vi "导入参数设置3.0.vi"(0 "路径":path) -> (7 "输出":T1)   [LabVIEW 2016]
uses:
  <vilib>/Utility/config.llb/Read Key (String).vi
  <vilib>/Utility/config.llb/Read Key (Double).vi
  <vilib>/Utility/config.llb/NI_LVConfig.lvlib
panel:
  in  "ESC":bool
  in  "OK":bool
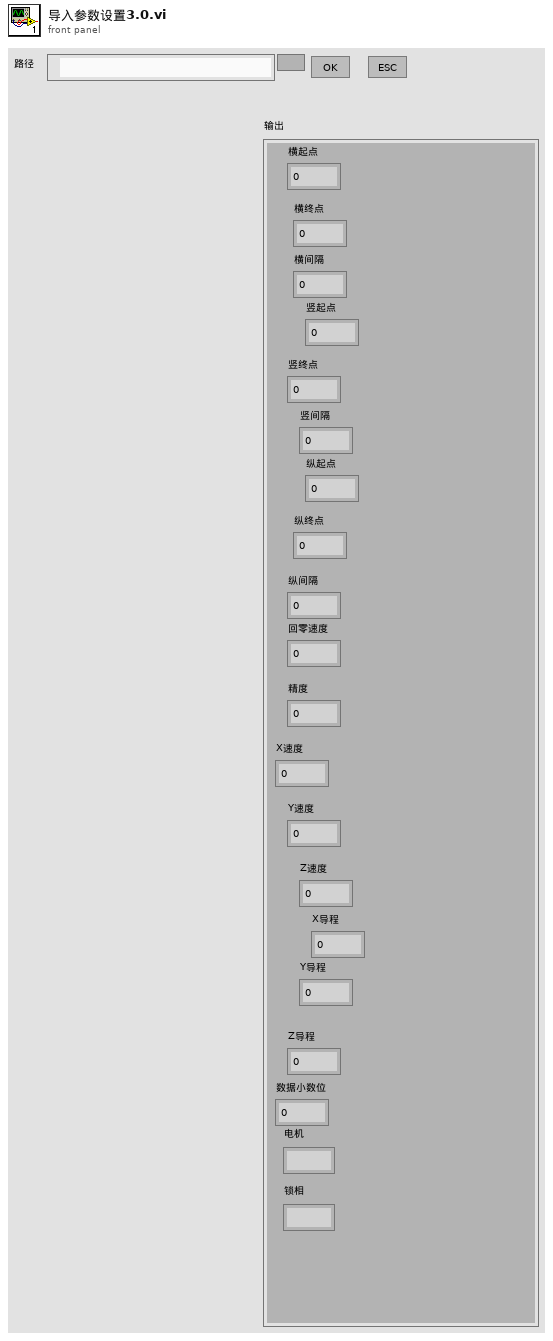
[diagram p1: front panel]
types:
  T1 = cluster{"横起点":dbl, "横终点":dbl, "横间隔":dbl, "竖起点":dbl, "竖终点":dbl, "竖间隔":dbl, "纵起点":dbl, "纵终点":dbl, "纵间隔":dbl, "回零速度":dbl, "精度":dbl, "X速度":dbl, "Y速度":dbl, "Z速度":dbl, "X导程":dbl, "Y导程":dbl, "Z导程":dbl, "数据小数位":dbl, "电机":string, "锁相":string}
  T2 = typedef "NI_LVConfig.lvlib/Config Data RefNum.ctl" = refnum<k1>
  T3 = cluster{"value":dbl, "value":dbl, "value":dbl, "value":dbl, "value":dbl, "value":dbl, "value":dbl, "value":dbl, "value":dbl, "value":dbl, "value":dbl, "value":dbl, "value":dbl, "value":dbl, "value":dbl, "value":dbl, "value":dbl, "value":dbl, "value":string, "value":string}
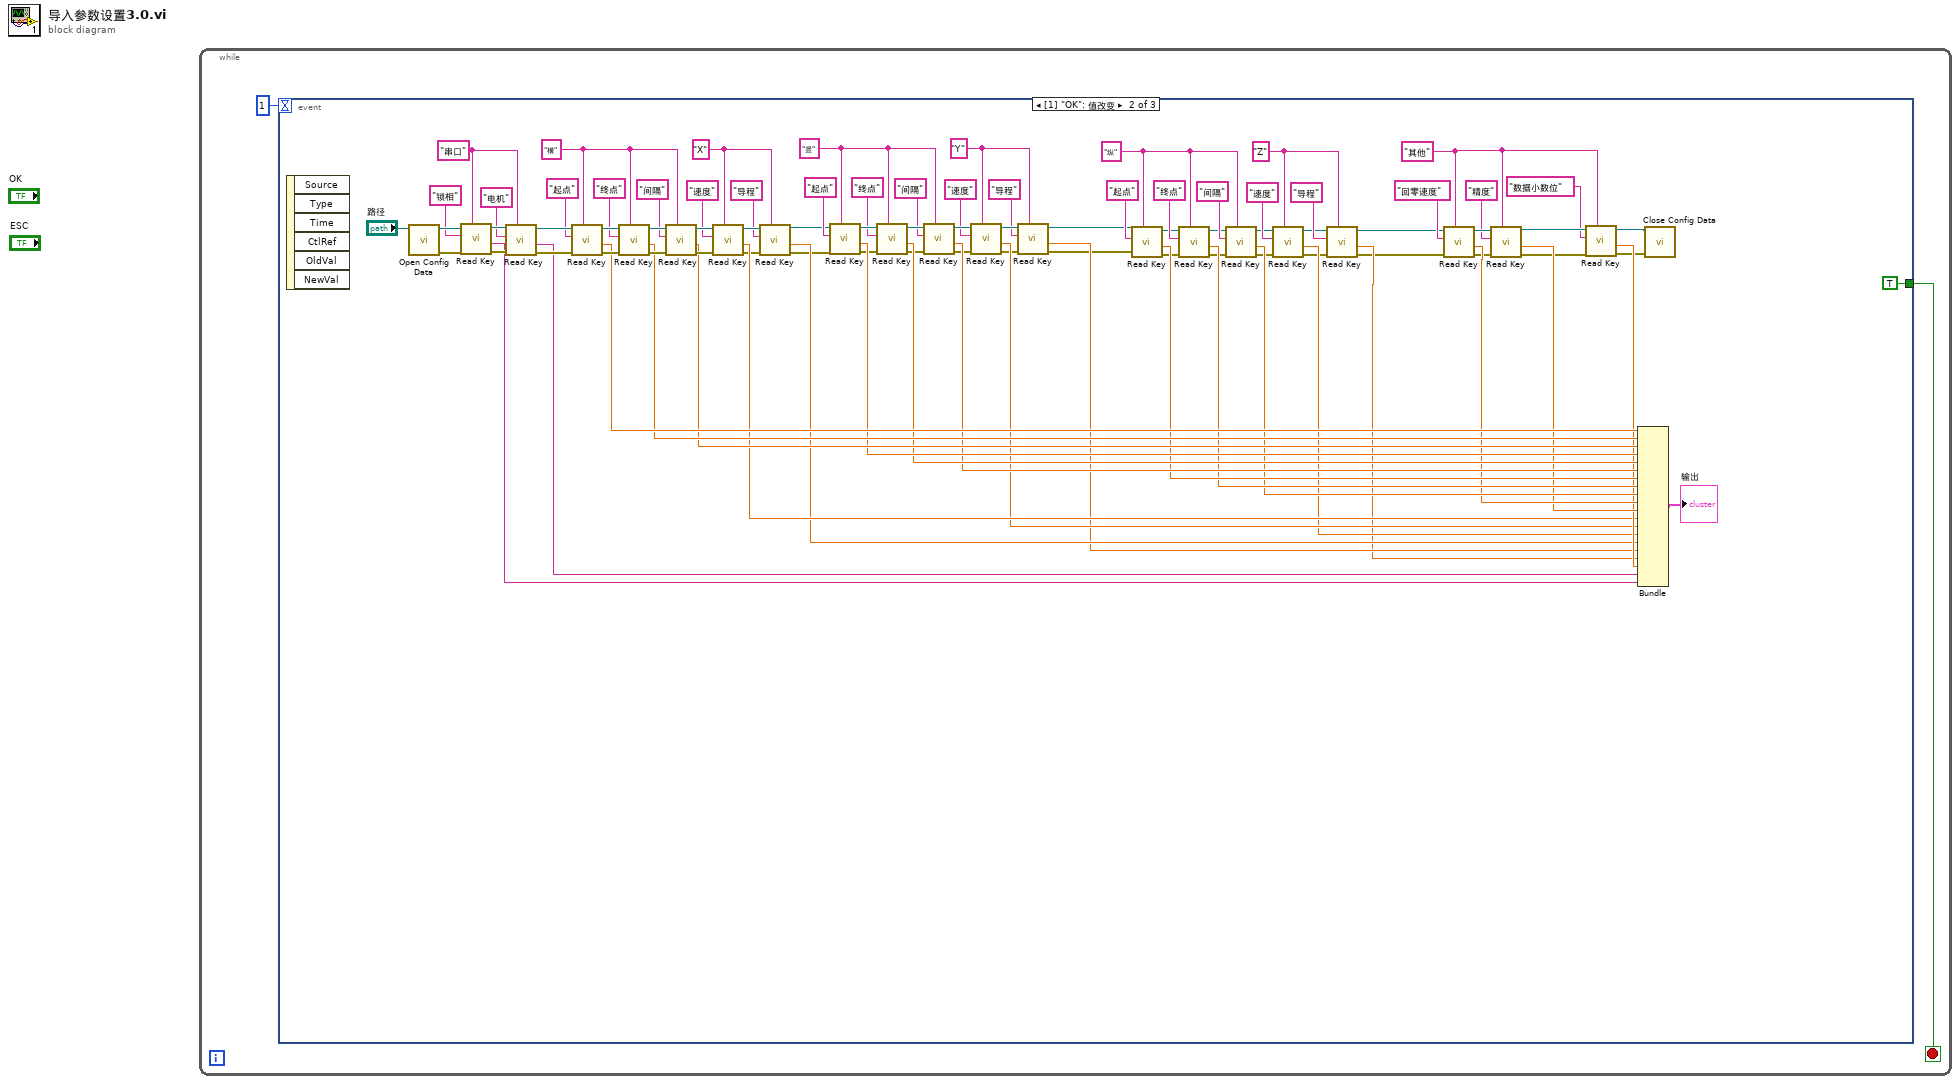
[diagram p0: block diagram]
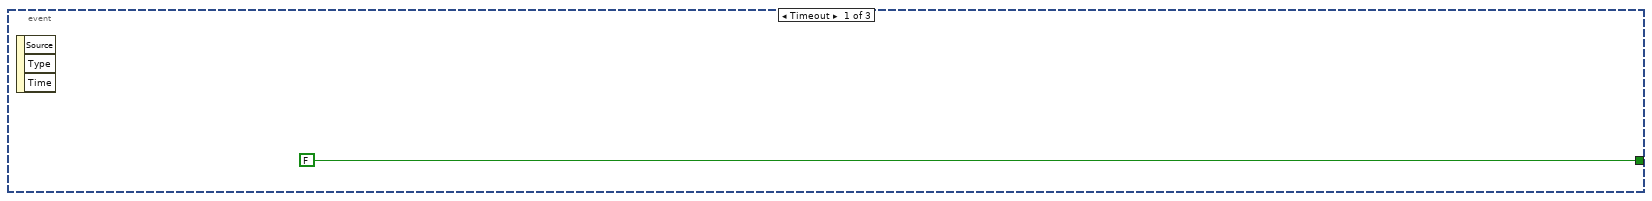
[diagram p2: hidden frame]
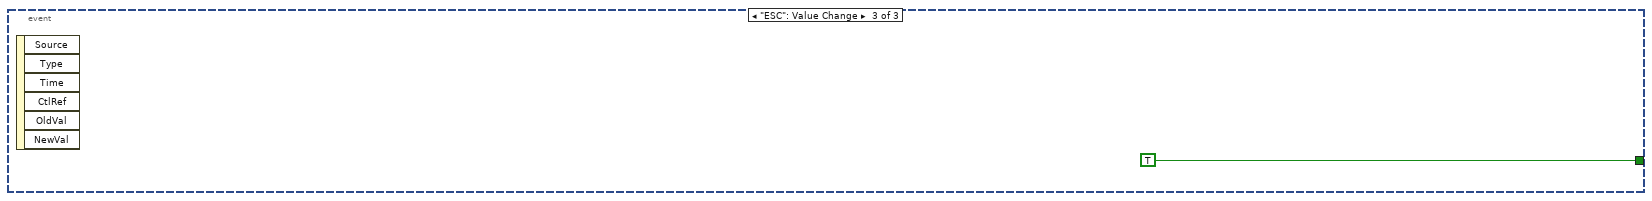
[diagram p3: hidden frame]
diagram:
  n1 = while {
    stop <- w1 stop-if-true
    n2 = event shown="[1] \"OK\": 值改变" {
      selector: _ -> [_ _ _]
      dyn-events: _ -> [_ _ _]
      timeout: 1 -> [_ _ _]
      tunnel: [FALSE TRUE TRUE] -> w1
      event Timeout {
        n3 = event-data() -> ()  [unwired: 1 in, 3 out]
      }
      event "OK": Value Change {
        w47 = "其他" ("section")
        w57 = "Y" ("section")
        w58 = "竖" ("section")
        w68 = "Z" ("section")
        w67 = "纵" ("section")
        w80 = "X" ("section")
        w82 = "横" ("section")
        w92 = "串口" ("section")
        n4 = event-data() -> ()  [unwired: 1 in, 6 out]
        n5 = call <vilib>:"Open Config Data.vi"("configuration file path"="路径") -> ("error out"=w87:errorcluster, "refnum"=w94:T2)  [unwired: 8 in, 1 out]
        n6 = call-poly <vilib>:"Read Key.vi"("section"=w92, "error in (no error)"=w87, "key"="锁相", "refnum"=w94) -> ("error out"=w86:errorcluster, "value"=w35:string, "refnum out"=w93:T2)  [unwired: 4 in, 1 out]
        n7 = call-poly <vilib>:"Read Key.vi"("section"=w92, "error in (no error)"=w86, "key"="电机", "refnum"=w93) -> ("error out"=w74:errorcluster, "value"=w36:string, "refnum out"=w81:T2)  [unwired: 4 in, 1 out]
        n8 = call-poly <vilib>:"Read Key.vi"("section"=w82, "error in (no error)"=w74, "key"="起点", "refnum"=w81) -> ("error out"=w91:errorcluster, "value"=w41:dbl, "refnum out"=w90:T2)  [unwired: 4 in, 1 out]
        n9 = call-poly <vilib>:"Read Key.vi"("section"=w82, "error in (no error)"=w91, "key"="终点", "refnum"=w90) -> ("error out"=w89:errorcluster, "value"=w40:dbl, "refnum out"=w88:T2)  [unwired: 4 in, 1 out]
        n10 = call-poly <vilib>:"Read Key.vi"("section"=w82, "error in (no error)"=w89, "key"="间隔", "refnum"=w88) -> ("error out"=w83:errorcluster, "value"=w39:dbl, "refnum out"=w85:T2)  [unwired: 4 in, 1 out]
        n11 = call-poly <vilib>:"Read Key.vi"("section"=w80, "error in (no error)"=w83, "key"="速度", "refnum"=w85) -> ("error out"=w19:errorcluster, "value"=w25:dbl, "refnum out"=w84:T2)  [unwired: 4 in, 1 out]
        n12 = call-poly <vilib>:"Read Key.vi"("section"=w80, "error in (no error)"=w19, "key"="导程", "refnum"=w84) -> ("error out"=w18:errorcluster, "value"=w22:dbl, "refnum out"=w51:T2)  [unwired: 4 in, 1 out]
        n13 = call-poly <vilib>:"Read Key.vi"("section"=w58, "error in (no error)"=w18, "key"="起点", "refnum"=w51) -> ("error out"=w17:errorcluster, "value"=w34:dbl, "refnum out"=w62:T2)  [unwired: 4 in, 1 out]
        n14 = call-poly <vilib>:"Read Key.vi"("section"=w58, "error in (no error)"=w17, "key"="终点", "refnum"=w62) -> ("error out"=w16:errorcluster, "value"=w33:dbl, "refnum out"=w61:T2)  [unwired: 4 in, 1 out]
        n15 = call-poly <vilib>:"Read Key.vi"("section"=w58, "error in (no error)"=w16, "key"="间隔", "refnum"=w61) -> ("error out"=w15:errorcluster, "value"=w32:dbl, "refnum out"=w60:T2)  [unwired: 4 in, 1 out]
        n16 = call-poly <vilib>:"Read Key.vi"("section"=w57, "error in (no error)"=w15, "key"="速度", "refnum"=w60) -> ("error out"=w14:errorcluster, "value"=w24:dbl, "refnum out"=w59:T2)  [unwired: 4 in, 1 out]
        n17 = call-poly <vilib>:"Read Key.vi"("section"=w57, "error in (no error)"=w14, "key"="导程", "refnum"=w59) -> ("error out"=w13:errorcluster, "value"=w21:dbl, "refnum out"=w50:T2)  [unwired: 4 in, 1 out]
        n18 = call-poly <vilib>:"Read Key.vi"("section"=w67, "error in (no error)"=w13, "key"="起点", "refnum"=w50) -> ("error out"=w12:errorcluster, "value"=w31:dbl, "refnum out"=w63:T2)  [unwired: 4 in, 1 out]
        n19 = call-poly <vilib>:"Read Key.vi"("section"=w67, "error in (no error)"=w12, "key"="终点", "refnum"=w63) -> ("error out"=w11:errorcluster, "value"=w30:dbl, "refnum out"=w64:T2)  [unwired: 4 in, 1 out]
        n20 = call-poly <vilib>:"Read Key.vi"("section"=w67, "error in (no error)"=w11, "key"="间隔", "refnum"=w64) -> ("error out"=w10:errorcluster, "value"=w29:dbl, "refnum out"=w65:T2)  [unwired: 4 in, 1 out]
        n21 = call-poly <vilib>:"Read Key.vi"("section"=w68, "error in (no error)"=w10, "key"="速度", "refnum"=w65) -> ("error out"=w9:errorcluster, "value"=w23:dbl, "refnum out"=w66:T2)  [unwired: 4 in, 1 out]
        n22 = call-poly <vilib>:"Read Key.vi"("section"=w68, "error in (no error)"=w9, "key"="导程", "refnum"=w66) -> ("error out"=w8:errorcluster, "value"=w20:dbl, "refnum out"=w43:T2)  [unwired: 4 in, 1 out]
        n23 = call-poly <vilib>:"Read Key.vi"("section"=w47, "error in (no error)"=w8, "key"="回零速度", "refnum"=w43) -> ("error out"=w7:errorcluster, "value"=w28:dbl, "refnum out"=w49:T2)  [unwired: 4 in, 1 out]
        n24 = call-poly <vilib>:"Read Key.vi"("section"=w47, "error in (no error)"=w7, "key"="精度", "refnum"=w49) -> ("error out"=w6:errorcluster, "value"=w27:dbl, "refnum out"=w48:T2)  [unwired: 4 in, 1 out]
        n25 = call-poly <vilib>:"Read Key.vi"("section"=w47, "error in (no error)"=w6, "key"="数据小数位", "refnum"=w48) -> ("error out"=w5:errorcluster, "value"=w26:dbl, "refnum out"=w42:T2)  [unwired: 4 in, 1 out]
        n26 = Bundle("value"=w41, "value"=w40, "value"=w39, "value"=w34, "value"=w33, "value"=w32, "value"=w31, "value"=w30, "value"=w29, "value"=w28, "value"=w27, "value"=w25, "value"=w24, "value"=w23, "value"=w22, "value"=w21, "value"=w20, "value"=w26, "value"=w36, "value"=w35) -> (→"输出":T3)  [unwired: 1 in]
        n27 = call <vilib>:"Close Config Data.vi"("error in (no error)"=w5, "refnum"=w42) -> ()  [unwired: 8 in, 2 out]
      }
      event "ESC": Value Change {
        n28 = event-data() -> ()  [unwired: 1 in, 6 out]
      }
    }
  }
